vi "Transmitter_Example_Image_Monokrom.vi"() -> ()   [LabVIEW 2018]
uses:
  <instrlib>/niUSRP/niUSRP Write Tx Data (CDB Cluster).vi
  <vilib>/picture/picture.llb/imagedata.ctl
panel:
  out "size(s) 2":i32[](array[numeric])
  out "output array":cdb[][](array[numeric])
  in  "OFDM Symbol":i32=20
  out "error out 2":errorcluster
  out "Frame Duration 2":dbl format="%#_6p"
  out "Waveform Graph 2":cluster{"t0":dbl, "dt":dbl, "Y":dbl[]}(graph)
  out "size(s)":i32
  out "output":i16[](array[numeric])
  out "0, 1":i16[][](array[numeric])
  out "1-bit pixmap":bool[][](array[boolean])
  out "new picture":picture
  out "image data":T1
  in  "path to BMP file":path
  out "bits":i32[](array[numeric])
  in  "Modulation parameter":T2
  out "Bits length":i32
  out "Frame Duration":dbl format="%#_6p"
  out "Waveform Graph":cluster{"t0":dbl, "dt":dbl, "Y":dbl[]}(graph)
  in  "stop":bool
  out "USRP CoercedParamters":T3={"coerced IQ rate"=100000.0, "coerced carrier frequency"=100000.0, "coerced gain"=0.0} {"coerced gain" format="%#_6f"; "coerced carrier frequency" format="%#_6p"; "coerced IQ rate" format="%#_6p"}
  out "error out":errorcluster
  in  "error in (no error)":errorcluster
  in  "USRP ControledParameters":T4={"active antenna"="TX1", "gain"=0.0, "carrier frequency"=915000000.0, "IQ rate"=1000000.0} {"IQ rate" format="%#_6p"; "carrier frequency" format="%#_6p"; "gain" format="%#_6f"}
  in  "device names":refnum<k15>="192.168.10.1"
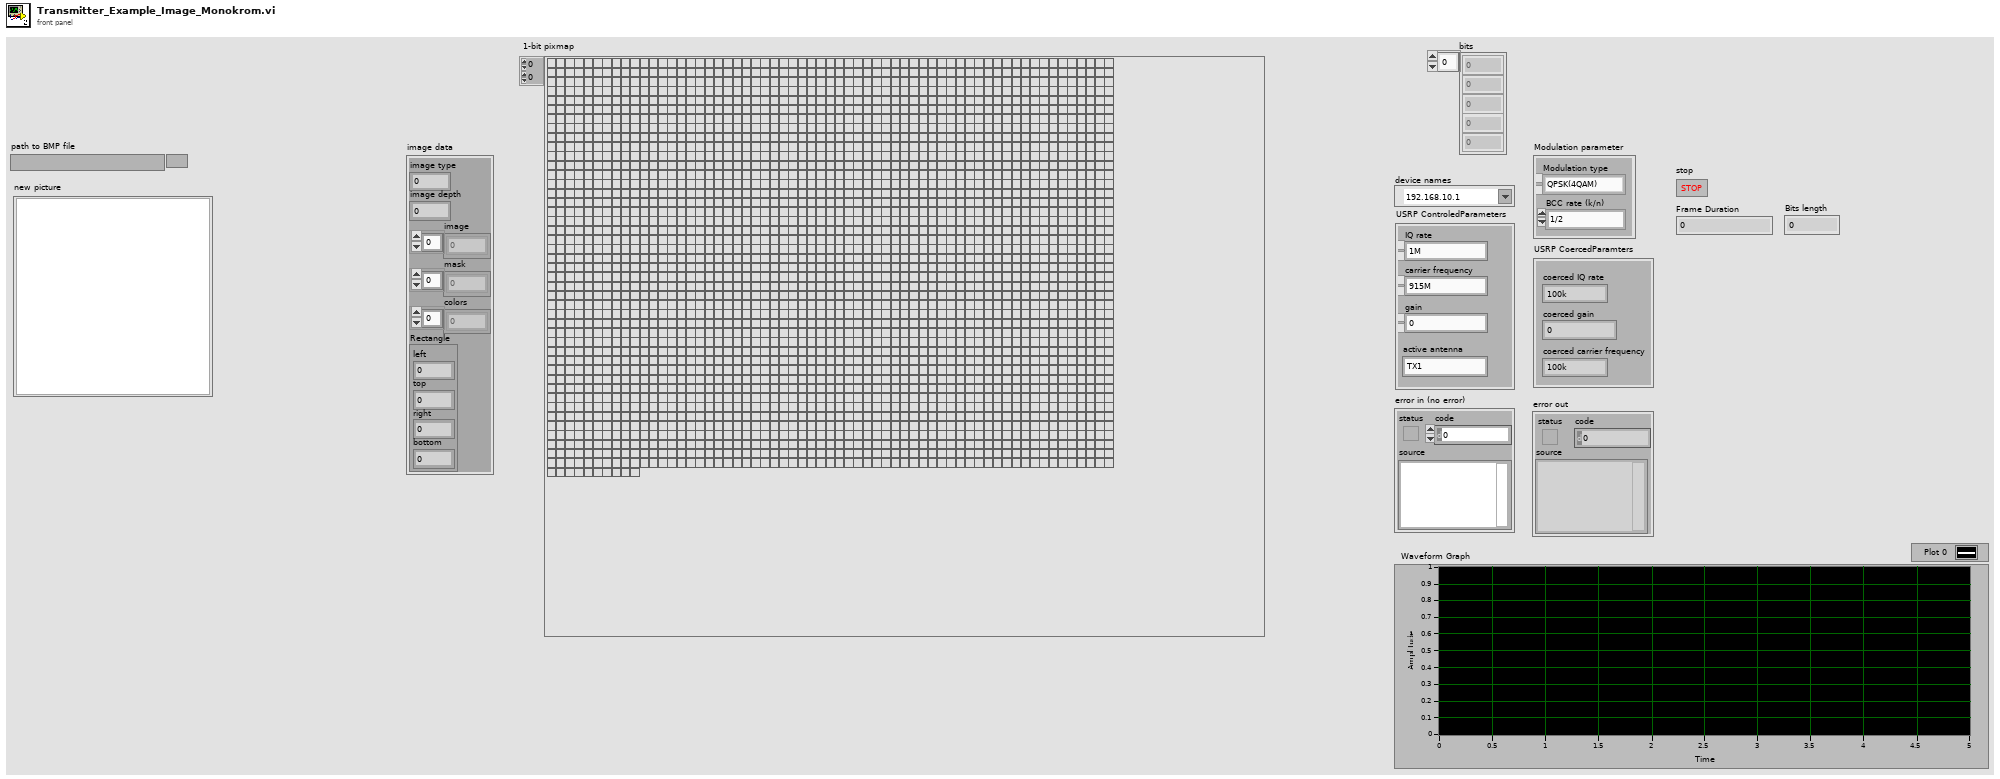
[diagram p1: front panel]
types:
  T1 = typedef "imagedata.ctl" = cluster{"image type":i32, "image depth":i32, "image":u8[], "mask":u8[], "colors":u32[], "Rectangle":cluster{"left":i16, "top":i16, "right":i16, "bottom":i16}}
  T2 = cluster{"Modulation type":enum16{"QPSK(4QAM)", "64QAM", "16QAM", "BPSK"}, "BCC rate (k/n)":enum16{"1/2", "2/3", "3/4"}}
  T3 = cluster{"coerced IQ rate":dbl, "coerced carrier frequency":dbl, "coerced gain":dbl}
  T4 = cluster{"active antenna":string, "gain":dbl, "carrier frequency":dbl, "IQ rate":dbl}
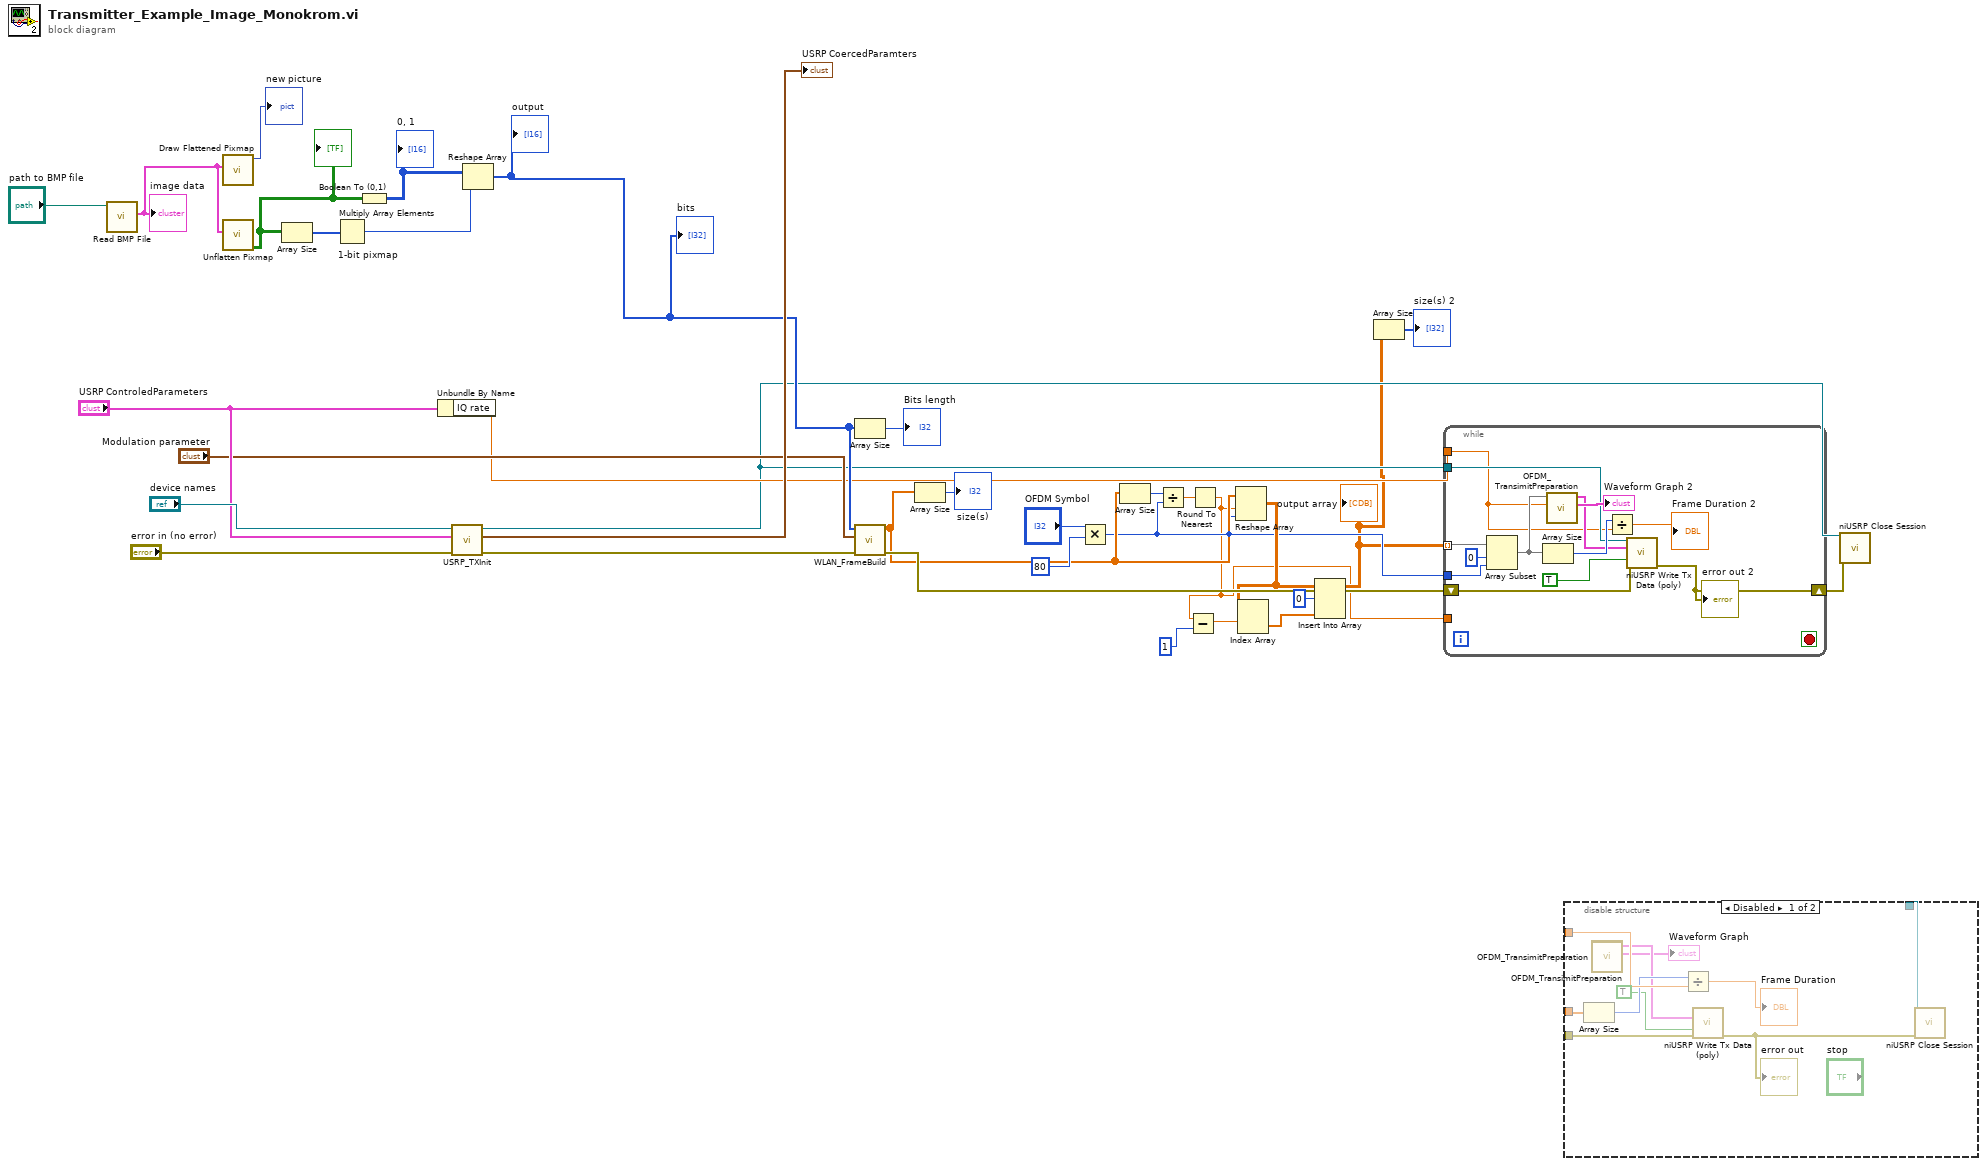
[diagram p0: block diagram]
diagram:
  n1 = call <vilib>:"Read BMP File.vi"("path to BMP file"="path to BMP file") -> ("image data"=w26:T1)  [unwired: 8 in, 2 out]
  "image data" <- w26
  n2 = call <vilib>:"Draw Flattened Pixmap.vi"("image data"=w26) -> ("new picture"=→"new picture":picture)  [unwired: 8 in]
  n3 = call <vilib>:"Unflatten Pixmap.vi"("image data"=w26) -> ("1-bit pixmap"=w24:bool[][])  [unwired: 4 in, 6 out]
  "1-bit pixmap" <- w24
  n4 = Array Size(array=w24) -> (size(s)=w25:i32[])
  n5 = Multiply Array Elements(1:w25) -> (0:w23:i32)
  n6 = Boolean To (0,1)(Boolean=w24) -> (0, 1=w22:i16[][])
  "0, 1" <- w22
  n7 = Unbundle By Name("USRP ControledParameters") -> ("IQ rate"=w18:dbl)
  n8 = call "USRP_TXInit.vi"("device names"="device names", "USRP ControledParameters"="USRP ControledParameters", "error in (no error)"="error in (no error)") -> ("session handle out"=w15:refnum<k15>, "USRP CoercedParamters"=→"USRP CoercedParamters":T3, "error out"=w29:errorcluster)  [unwired: 5 in]
  n9 = Reshape Array(w22, w23) -> (w21:i16[])
  "bits" <- w21
  "output" <- w21
  n10 = Array Size(array=w21) -> (size(s)=→"Bits length":i32)
  n11 = call "WLAN_FrameBuild.vi"("error in (no error)"=w29, "Modulation parameter"="Modulation parameter", "data in"=w21) -> ("error out"=w17:errorcluster, "output array"=w10:cdb[])  [unwired: 4 in, 3 out]
  n12 = Array Size(array=w10) -> (size(s)=→"size(s)":i32)
  n13 = Multiply(x="OFDM Symbol", y=80) -> (x*y=w6:i32)
  n14 = Array Size(array=w10) -> (size(s)=w14:i32)
  n15 = Divide(x=w14, y=w6) -> (x/y=w13:dbl)
  n16 = Round To Nearest(number=w13) -> (nearest integer value=w1:dbl)
  n17 = Subtract(x=w1, y=1) -> (x-y=w4:dbl)
  n18 = Reshape Array(w10, w1, w6) -> (w9:cdb[][])
  n19 = Index Array(array=w9, index (row)=w4) -> (element=w8:cdb[])  [unwired: 1 in]
  n20 = Insert Into Array(array=w9, index (row)=0, new element=w8) -> (w3:cdb[][])  [unwired: 1 in]
  "output array" <- w3
  n21 = Array Size(array=w3) -> (size(s)=→"size(s) 2":i32[])
  n22 = while {
    tunnel: w3 -> [w47] mode=indexing
    tunnel: w6 -> [w45]
    tunnel: w18 -> [w35]
    shift-right: [w37] -> w16
    shift-left: w17 -> [w38]
    tunnel: w15 -> [w36]
    tunnel: w1 -> [_]
    stop <- _ stop-if-true
    n23 = Array Subset(array=w47, index=0, length=w45) -> (w44:cdb[])
    n24 = Array Size(array=w44) -> (size(s)=w43:i32)
    n25 = call "OFDM_TransimitPreparation.vi"("IQ rate"=w35, "array"=w44) -> ("output cluster 2"=→"Waveform Graph 2":cluster{"t0":dbl, "dt":dbl, "Y":cdb[]}, "output cluster"=w41:cluster{"t0":dbl, "dt":dbl, "Y":cdb[]})  [unwired: 8 in]
    n26 = Divide(x=w43, y=w35) -> (x/y=→"Frame Duration 2":dbl)
    n27 = call-poly <instrlib>:"niUSRP Write Tx Data (poly).vi"("session handle"=w36, "data"=w41, "end of data?"=TRUE, "error in (no error)"=w38) -> ("error out"=w37:errorcluster)  [unwired: 10 in, 1 out]
    "error out 2" <- w37
  }
  n28 = disable-structure shown="Disabled" {
    disable-tunnel: _ -> [w58 _]
    disable-tunnel: _ -> [w57 _]
    disable-tunnel: _ -> [w52 _]
    disable-tunnel: _ -> [w51 _]
    frame Disabled {
      n29 = Array Size(array=w51) -> (size(s)=w55:i32)
      n30 = call "OFDM_TransimitPreparation.vi"() -> ()  [unwired: 10 in, 2 out]
      n31 = call "OFDM_TransimitPreparation.vi"() -> ("output cluster 2"=→"Waveform Graph":cluster{"t0":dbl, "dt":dbl, "Y":cdb[]}, "output cluster"=w53:cluster{"t0":dbl, "dt":dbl, "Y":cdb[]})  [unwired: 10 in]
      n32 = Divide(x=w55, y=w58) -> (x/y=→"Frame Duration":dbl)
      n33 = call-poly <instrlib>:"niUSRP Write Tx Data (poly).vi"("data"=w53, "end of data?"=TRUE, "error in (no error)"=w52) -> ("session handle"=w48:refnum<k15>, "error out"=w56:errorcluster)  [unwired: 10 in, 1 out]
      "error out" <- w56
      n34 = call <instrlib>:"niUSRP Close Session.vi"("session handle"=w57, "error in (no error)"=w56) -> ()  [unwired: 13 in, 1 out]
    }
    frame Enabled {
    }
  }
  n35 = call <instrlib>:"niUSRP Close Session.vi"("session handle"=w15, "error in (no error)"=w16) -> ()  [unwired: 13 in, 1 out]
